vi "OAT Polar Calculate Orbit Coordinats for Picture.vi"(6 "polar attributes":T1 {"minimum" format="%.2f"; "maximum" format="%.2f"}, 10 "grid measurements":T3 {"end angle" format="%.2f"; "start angle" format="%.2f"; "scale factors"."b" format="%.2f"; "scale factors"."a" format="%.2f"}, 11 "?":T2 {"Location"."phase" format="%.2f"; "Location"."mag" format="%.2f"}) -> (2 "position":cluster{"x":i16, "y":i16}, 3 "Name":string)   [LabVIEW 2017]
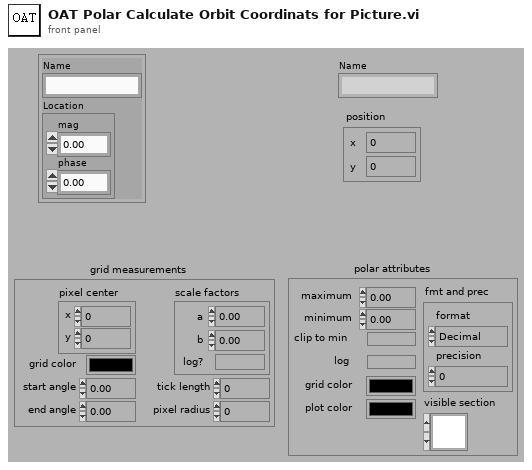
[diagram p1: front panel]
types:
  T1 = cluster{"maximum":dbl, "minimum":dbl, "clip to min":bool, "log":bool, "grid color":u32, "plot color":u32, "fmt and prec":cluster{"format":enum8{"Decimal", "Scientific", "Engineering", "Binary", "Octal", "Hex"}, "precision":u8}, "visible section":u16}
  T2 = cluster{"Name":string, "Location":cluster{"mag":dbl, "phase":dbl}}
  T3 = cluster{"pixel center":cluster{"x":i16, "y":i16}, "scale factors":cluster{"a":dbl, "b":dbl, "log?":bool}, "grid color":u32, "start angle":dbl, "end angle":dbl, "tick length":i16, "pixel radius":i32}
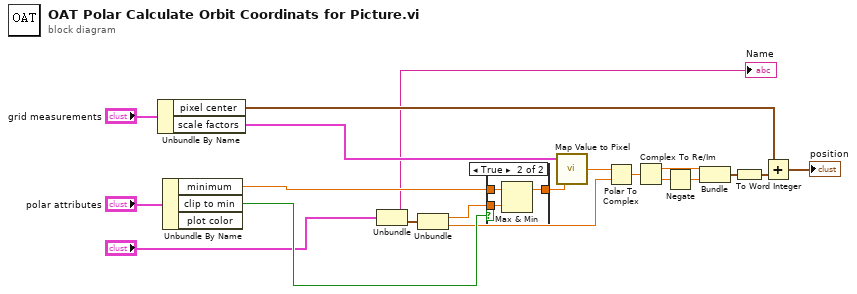
[diagram p0: block diagram]
diagram:
  n1 = Unbundle By Name("grid measurements") -> ("pixel center"=w17:cluster{"x":i16, "y":i16}, "scale factors"=w18:cluster{"a":dbl, "b":dbl, "log?":bool})
  n2 = Unbundle By Name("polar attributes") -> ("minimum"=w16:dbl, "clip to min"=w15:bool)  [unwired: 1 out]
  n3 = Unbundle("?") -> ("Name"=→"Name":string, "Location"=w4:cluster{"mag":dbl, "phase":dbl})
  n4 = Unbundle(w4) -> ("mag"=w3:dbl, "phase"=w2:dbl)
  n5 = case shown="True" w15 {
    tunnel: w3 -> [w21 w24]
    tunnel: [w21 w23] -> w5
    tunnel: w16 -> [_ w22]
    frame False {
    }
    frame True {
      n6 = Max & Min(x=w22, y=w24) -> (max(x,y)=w23:dbl)  [unwired: 1 out]
    }
  }
  n7 = call <vilib>:"Map Value to Pixel.vi"("x"=w5, "scale factors"=w18) -> ("pixel"=w6:dbl)  [unwired: 1 in]
  n8 = Polar To Complex(1:w2, 2:w6) -> (0:w12:cdb)
  n9 = Complex To Re/Im(x + iy=w12) -> (x=w10:dbl, y=w9:dbl)
  n10 = Negate(x=w9) -> (-x=w7:dbl)
  n11 = Bundle(w10, w7) -> (w11:cluster{dbl, dbl})  [unwired: 1 in]
  n12 = To Word Integer(number=w11) -> (16bit integer=w8:cluster{i16, i16})
  n13 = Add(x=w17, y=w8) -> (x+y=→"position":cluster{i16, i16})
